vi "Main.vi"(8 "error in":errorcluster, 11 "ArduinoOperator in":refnum<class "ArduinoOperator.lvclass">) -> (0 "error out":errorcluster, 3 "ArduinoOperator out":refnum<class "ArduinoOperator.lvclass">)   [LabVIEW 2018, in "ArduinoOperator.lvclass"]
doc: "The Queued Message Handler of a Worker."
uses:
  ArduinoOperator.lvclass
  Initialization Data.ctl
  <vilib>/addons/_Workers/Library/Classes/Worker/Worker.lvclass
  <vilib>/addons/_Workers/Library/Classes/Message/Message.lvclass
  <vilib>/addons/_Workers/Library/Classes/Message/Enqueue Message to Self v2.vi
  <vilib>/MakerHub/LINX/LMH-LINX.lvlib
  <vilib>/MakerHub/LINX/Public/Utilities/Open Serial.vi
  <vilib>/MakerHub/LINX/Public/Peripherals/Digital/Digital Read 1 Chan.vi
  <vilib>/MakerHub/LINX/Public/Peripherals/Analog/Analog Read 1 Chan.vi
  <vilib>/MakerHub/LINX/Public/Peripherals/Digital/Digital Write 1 Chan.vi
  <vilib>/addons/_Workers/Library/Classes/Message Queue/Message Queue.lvclass
  <vilib>/addons/_Workers/Library/Classes/Message/Priority.ctl
  Timer/Timer.lvclass
  <vilib>/addons/_Workers/Library/Classes/Message/Enqueue Message to Queue.vi
  C:/Program Files (x86)/National Instruments/LabVIEW 2022/vi.lib/addons/_Workers/Library/Classes/Worker/Worker.lvclass
  C:/Program Files (x86)/National Instruments/LabVIEW 2022/vi.lib/addons/_Workers/Library/Classes/Workers Object/Workers Object.lvclass
  <vilib>/addons/_Workers/Library/Classes/Message/Enqueue Message to Self v2 - Silent Mode - Array.vi
panel:
  out "Target":bool
  in  "TimerON":bool
  in  "TimerCount(S)":i32=1
  out "Loop Rate (Hz)":u32
  in  "Close":bool
  in  "Link":bool
  in  "AI Channel":u8
  out "Analog Data":dbl(graph)
  in  "DI Channel":u8=2
  out "DI Value":bool
  in  "DO Value":bool
  in  "DO Channel":u8=3
  in  "Serial Port":refnum<visa-resource-name>
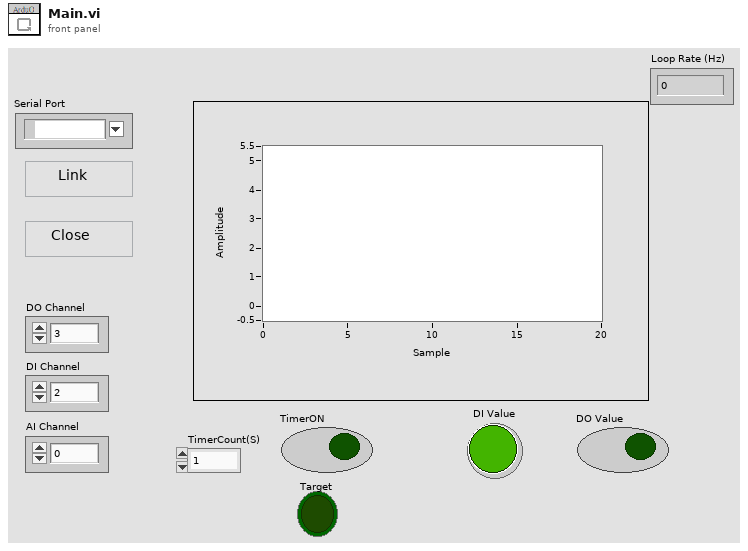
[diagram p1: front panel]
types:
  T1 = typedef "ArduinoOperator.lvclass/Initialization Data.ctl" = cluster{"String":string}
  T2 = typedef "Workers.lvlib/Message.lvclass/Priority.ctl" = enum16{"Low", "Normal", "High"}
  T3 = typedef "Workers.lvlib/Case Label.ctl" = string
  T4 = cluster{"Message Queue out":refnum<class "Message Queue.lvclass">, "Case Label":T3}
  T5 = typedef "LMH-LINX.lvlib/LINX Ref.ctl" = cluster{"IO":T6, "Interface":T7, "LINX Device Config":T8}
  T6 = typedef "LMH-LINX.lvlib/Platform.ctl" = enum16{"Remote", "Local"}
  T7 = typedef "LMH-LINX.lvlib/Interface.ctl" = enum16{"Serial", "TCP"}
  T8 = typedef "LMH-LINX.lvlib/Device.lvlib/LINX Device Config.ctl" = cluster{"Interface":T7, "COM Port":refnum<visa-resource-name>, "TCP Configuration":T9, "Device Family":u8, "Device ID":u8, "Device Name":string, "TCP Ref":refnum<k5>, "Channels":T10}
  T9 = typedef "LMH-LINX.lvlib/Device.lvlib/TCP Config.ctl" = cluster{"IP Address":string, "Port":u16}
  T10 = typedef "LMH-LINX.lvlib/Channels.ctl" = cluster{"DI":u8[], "DO":u8[], "AI":u8[], "AO":u8[], "PWM":u8[], "QE":u8[], "UART":u8[], "I2C 2":u8[], "SPI":u8[], "CAN":u8[], "Servo":u8[], "AI Ref (V)":dbl, "AI Resolution (Bits)":u8, "AO Ref (V)":dbl, "AO Resolution (Bits)":u8}
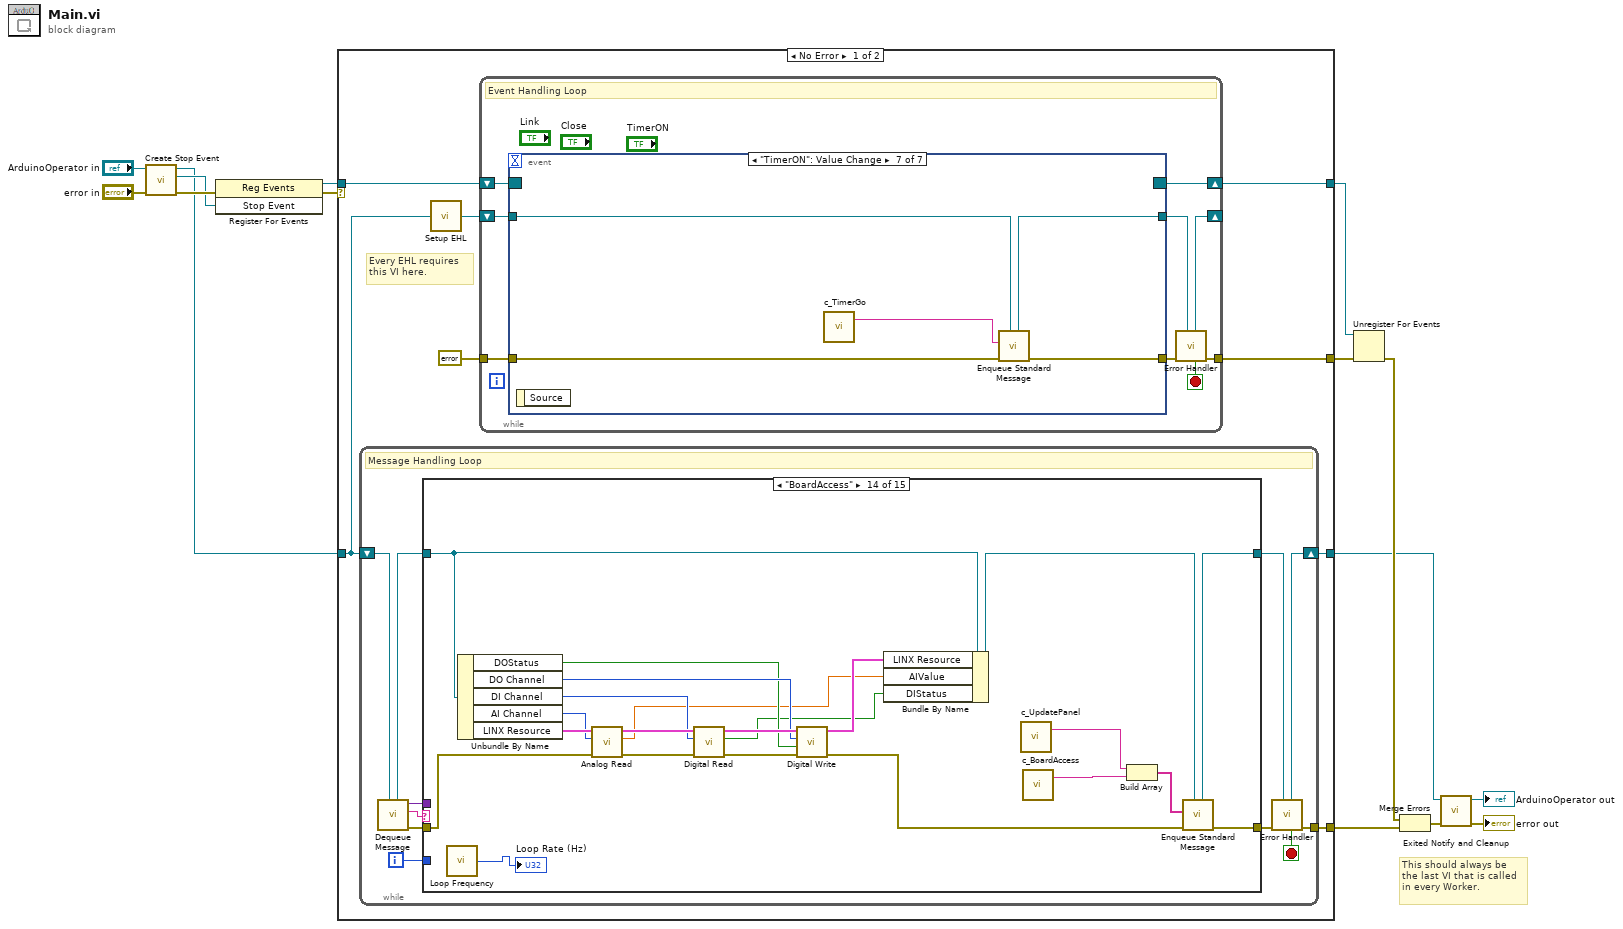
[diagram p0: block diagram]
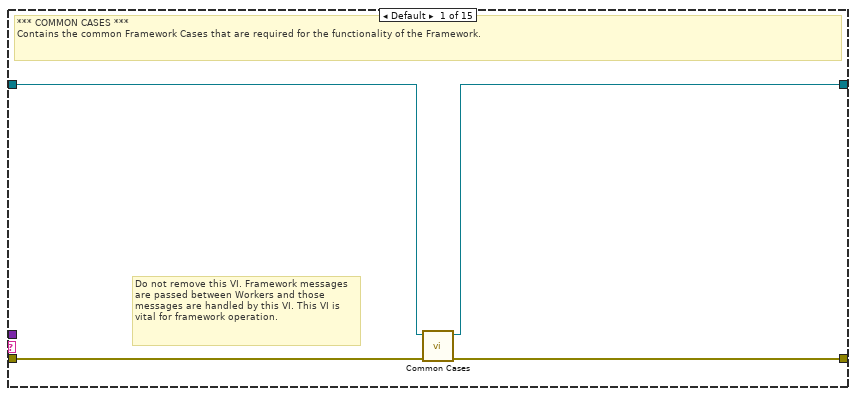
[diagram p2: hidden frame]
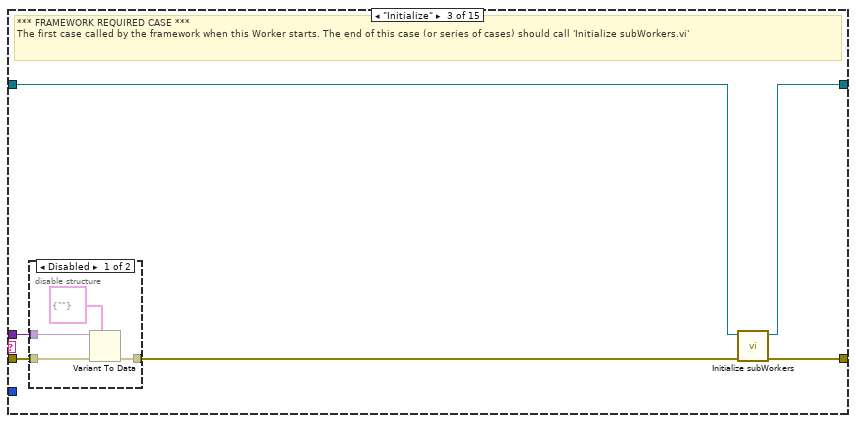
[diagram p4: hidden frame]
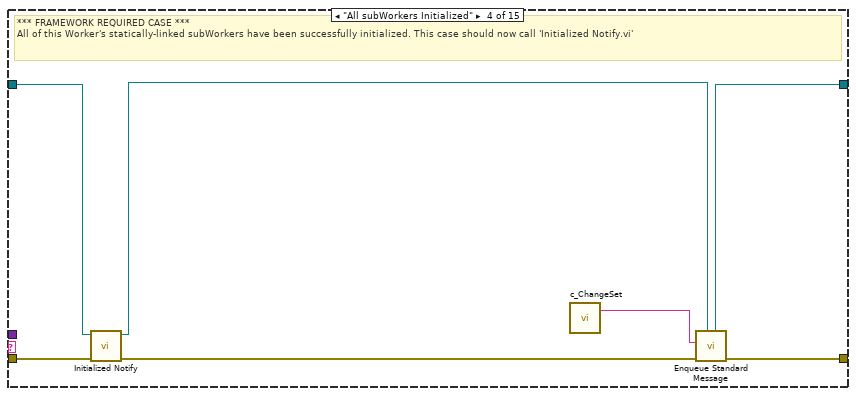
[diagram p6: hidden frame]
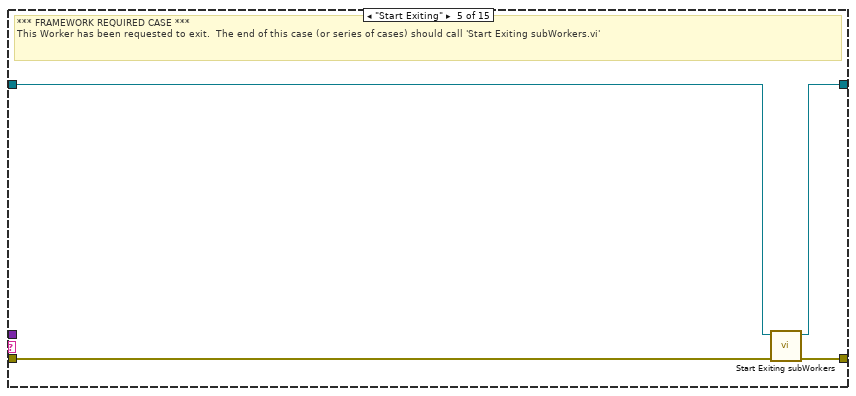
[diagram p7: hidden frame]
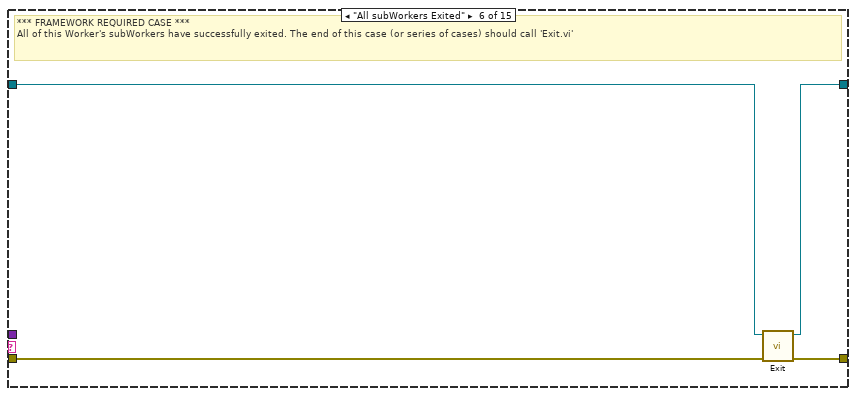
[diagram p8: hidden frame]
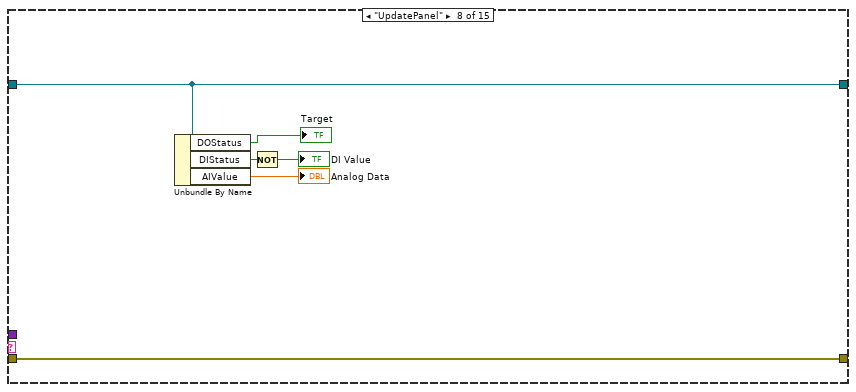
[diagram p10: hidden frame]
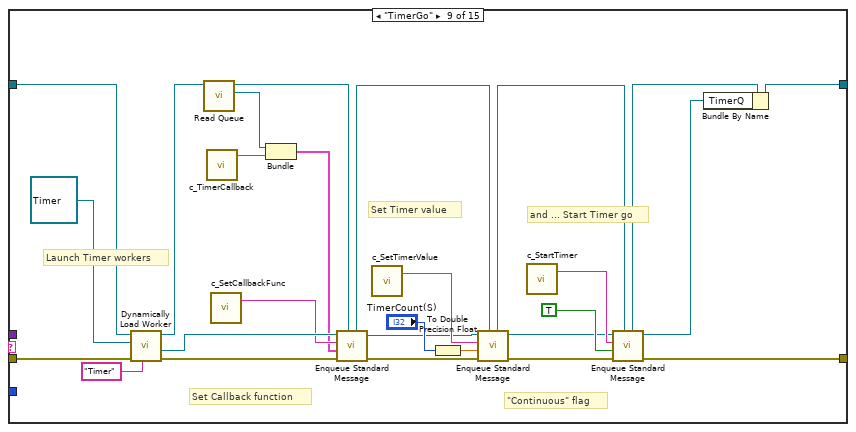
[diagram p11: hidden frame]
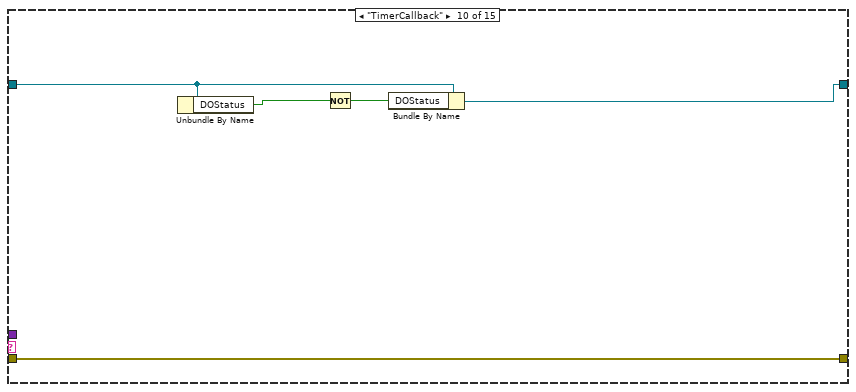
[diagram p12: hidden frame]
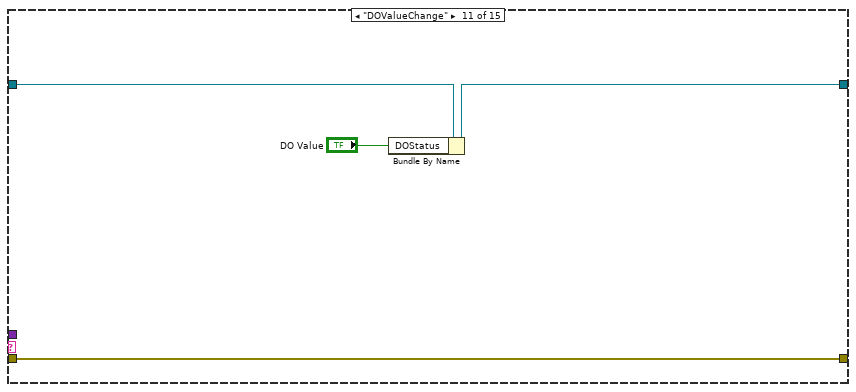
[diagram p13: hidden frame]
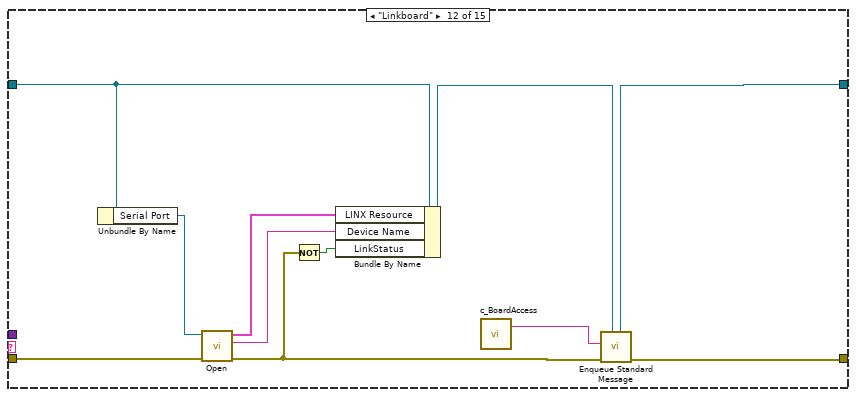
[diagram p14: hidden frame]
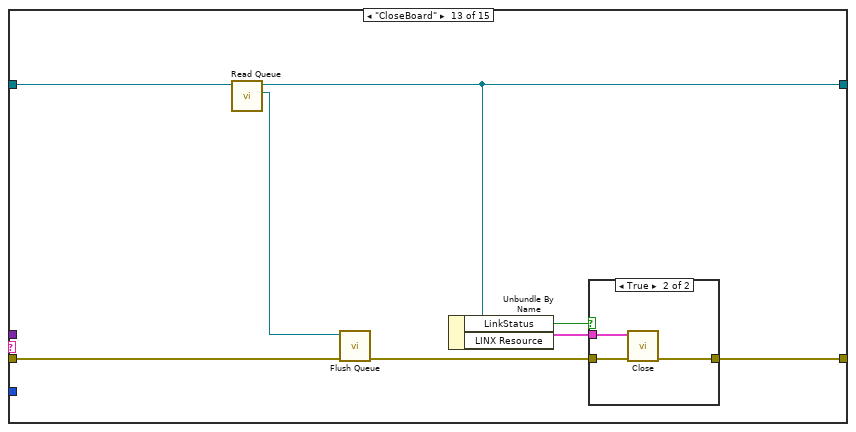
[diagram p15: hidden frame]
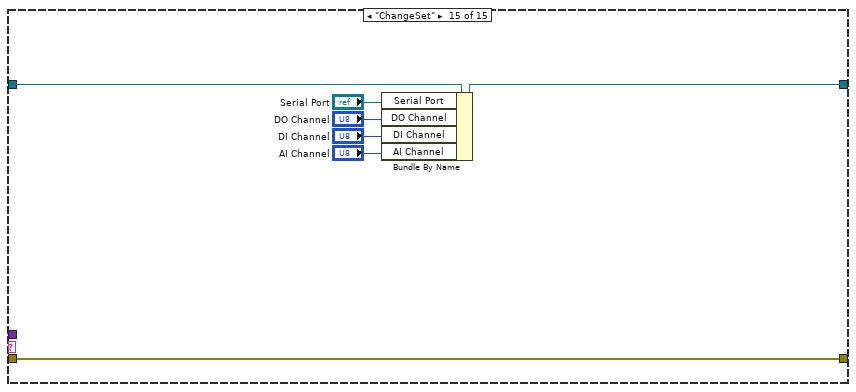
[diagram p17: hidden frame]
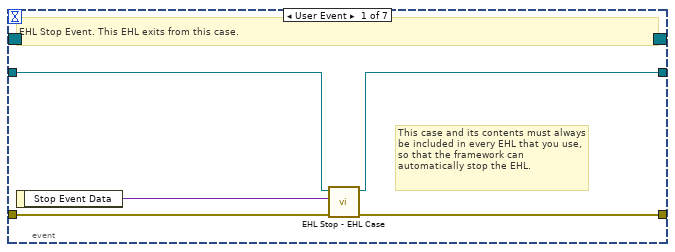
[diagram p18: hidden frame]
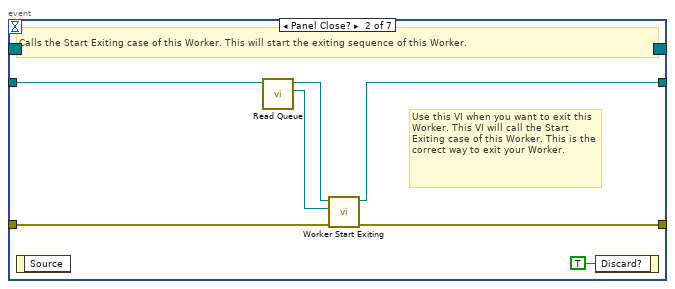
[diagram p19: hidden frame]
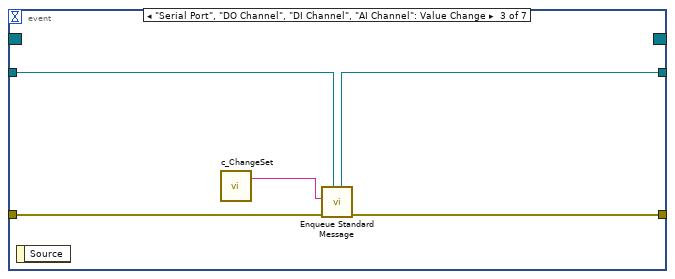
[diagram p20: hidden frame]
diagram:
  # "This should always be the last VI that is called in every Worker."
  n1 = call-dynamic "Create Stop Event.vi"("error in"="error in", "Worker"="ArduinoOperator in") -> ("error out"=w10:errorcluster, "Stop Event"=w7:refnum<user-event>, "Worker out"=w4:refnum<class "ArduinoOperator.lvclass">)  [unwired: 7 in]
  n2 = register-events(error in=w10, w7) -> (reference out=w9:refnum<event-registration>, error out=w1:errorcluster)  [unwired: 1 in]
  n3 = case shown="No Error" w1 {
    tunnel: w4 -> [w18 w211]
    tunnel: [w16 w212] -> w8
    tunnel: w9 -> [w23 w213]
    tunnel: [w20 w214] -> w14
    tunnel: [w22 w213] -> w13
    tunnel: [w17 w210] -> w11
    selector: w1 -> [_ w214]
    frame No Error {
      # "Every EHL requires\nthis VI here."
      n4 = while {
        shift-right: [w32] -> w17
        shift-left: w18 -> [w34]
        tunnel: [w33] -> w16
        i -> [w24]
        stop <- w25 stop-if-true
        # "Message Handling Loop"
        n5 = call-dynamic "Dequeue Message.vi"("Worker"=w34) -> ("error out"=w31:errorcluster, "Case out"=w26:string, "Data out"=w27:variant, "Worker out"=w29:refnum<class "ArduinoOperator.lvclass">)  [unwired: 6 in, 1 out]
        n6 = case "Worker MHL Case Structure (DO NOT CHANGE LABEL NAME)" shown="\"BoardAccess\"" w26 {
          tunnel: w31 -> [w38 w39 w44 w57 w59 w66 w67 w74 w101 w106 w110 w121 w125 w148 w162]
          tunnel: [w37 w39 w46 w55 w62 w65 w67 w74 w93 w106 w110 w113 w126 w138 w162] -> w30
          tunnel: w29 -> [w36 w40 w43 w58 w60 w64 w68 w73 w99 w105 w109 w120 w129 w152 w161]
          tunnel: [w35 w40 w45 w53 w61 w63 w68 w73 w76 w102 w108 w114 w123 w140 w160] -> w28
          tunnel: w27 -> [_ _ w41 _ _ _ _ _ _ _ _ _ _ _ _]
          tunnel: w24 -> [_ _ _ _ _ _ _ _ _ _ _ _ _ _ _]
          frame Default {
            # "Do not remove this VI. Framework messages are passed between Workers and those messages are handled by this VI. This VI is vital for framework operation."
            # "*** COMMON CASES ***\nContains the common Framework Cases that are required for the functionality of the Framework."
            n7 = call-dynamic "Common Cases.vi"("error in"=w38, "Worker in"=w36) -> ("error out"=w37:errorcluster, "Worker out"=w35:refnum<class "ArduinoOperator.lvclass">)  [unwired: 8 in]
          }
          frame "------ FRAMEWORK REQUIRED CASES ------" {
            # "Start of Framework Required Cases"
          }
          frame "Initialize" {
            # "*** FRAMEWORK REQUIRED CASE ***\nThe first case called by the framework when this Worker starts. The end of this case (or series of cases) should call 'Initialize subWorkers.vi'"
            n8 = disable-structure shown="Disabled" {
              disable-tunnel: w44 -> [w50 w51]
              disable-tunnel: [w49 w51] -> w42
              disable-tunnel: w41 -> [w48 _]
              frame Disabled {
                n9 = Variant To Data(error in=w50, type=T1 {"String"=""} ("Initialization Data"), Variant=w48) -> (error out=w49:errorcluster)  [unwired: 1 out]
              }
              frame Enabled {
              }
            }
            n10 = call-dynamic "Initialize subWorkers.vi"("error in"=w42, "Worker"=w43) -> ("error out"=w46:errorcluster, "dup Worker out"=w45:refnum<class "ArduinoOperator.lvclass">)  [unwired: 8 in]
          }
          frame "All subWorkers Initialized" {
            # "*** FRAMEWORK REQUIRED CASE ***\nAll of this Worker's statically-linked subWorkers have been successfully initialized. This case should now call 'Initialized Notify.vi'"
            n11 = call-dynamic "Initialized Notify.vi"("error in"=w57, "Worker"=w58) -> ("error out"=w56:errorcluster, "dup Worker out"=w54:refnum<class "ArduinoOperator.lvclass">)  [unwired: 8 in]
            n12 = call "c_ChangeSet.vi"() -> ("Case Label"=w52:T3)  [unwired: 1 in]
            n13 = call-poly <vilib>:"Enqueue Standard Message.vi"("Worker"=w54, "error in"=w56, "Case Label"=w52) -> ("error out"=w55:errorcluster, "dup Worker out"=w53:refnum<class "ArduinoOperator.lvclass">)  [unwired: 7 in]
          }
          frame "Start Exiting" {
            # "*** FRAMEWORK REQUIRED CASE ***\nThis Worker has been requested to exit.  The end of this case (or series of cases) should call 'Start Exiting subWorkers.vi'"
            n14 = call-dynamic "Start Exiting subWorkers.vi"("error_in"=w59, "Worker"=w60) -> ("error out"=w62:errorcluster, "dup Worker out"=w61:refnum<class "ArduinoOperator.lvclass">)  [unwired: 8 in]
          }
          frame "All subWorkers Exited" {
            # "*** FRAMEWORK REQUIRED CASE ***\nAll of this Worker's subWorkers have successfully exited. The end of this case (or series of cases) should call 'Exit.vi'"
            n15 = call-dynamic "Exit.vi"("error_in"=w66, "Worker"=w64) -> ("error out"=w65:errorcluster, "dup Worker out"=w63:refnum<class "ArduinoOperator.lvclass">)  [unwired: 8 in]
          }
          frame "-----------------------------------------------" {
            # "End of Framework Required Cases"
          }
          frame "UpdatePanel" {
            n16 = Unbundle By Name(w73) -> ("DOStatus"=→"Target":bool, "DIStatus"=w72:bool, "AIValue"=→"Analog Data":dbl)
            n17 = Not(x=w72) -> (.not. x?=→"DI Value":bool)
          }
          frame "TimerGo" {
            # "\"Continuous\" flag"
            # "and ... Start Timer go"
            # "Set Timer value"
            # "Set Callback function"
            # "Launch Timer workers"
            n18 = call <vilib>:"Dynamically Load Worker.vi"("Worker Alias"="Timer", "error in"=w101, "Worker to Dynamically Load"=refnum<class "Timer.lvclass"> refnum ("Timer.lvclass"), "Worker"=w99) -> ("error out"=w100:errorcluster, "Message Queue out"=w84:refnum<class "Message Queue.lvclass">, "dup Worker out"=w86:refnum<class "ArduinoOperator.lvclass">)  [unwired: 4 in, 1 out]
            n19 = call <vilib>:"Read Queue.vi"("Worker"=w86) -> ("Message Queue out"=w79:refnum<class "Message Queue.lvclass">, "dup Worker out"=w81:refnum<class "ArduinoOperator.lvclass">)  [unwired: 9 in]
            n20 = call "c_TimerCallback.vi"() -> ("Case Label"=w80:T3)  [unwired: 1 in]
            n21 = call "c_SetCallbackFunc.vi"() -> ("Case Label"=w82:T3)  [unwired: 1 in]
            n22 = Bundle("Message Queue out"=w79, "Case Label"=w80) -> (w78:T4)  [unwired: 1 in]
            n23 = call-poly <vilib>:"Enqueue Standard Message.vi"("Worker"=w81, "error in"=w100, "Data"=w78, "Case Label"=w82, "Message Queue"=w84) -> ("error out"=w87:errorcluster, "dup Message Queue out"=w83:refnum<class "Message Queue.lvclass">, "dup Worker out"=w85:refnum<class "ArduinoOperator.lvclass">)  [unwired: 4 in]
            n24 = call "c_SetTimerValue.vi"() -> ("Case Label"=w96:T3)  [unwired: 1 in]
            n25 = To Double Precision Float(number="TimerCount(S)") -> (double precision float=w94:dbl)
            n26 = call-poly <vilib>:"Enqueue Standard Message.vi"("Worker"=w85, "error in"=w87, "Data"=w94, "Case Label"=w96, "Message Queue"=w83) -> ("error out"=w97:errorcluster, "dup Message Queue out"=w77:refnum<class "Message Queue.lvclass">, "dup Worker out"=w92:refnum<class "ArduinoOperator.lvclass">)  [unwired: 4 in]
            n27 = call "c_StartTimer.vi"() -> ("Case Label"=w90:T3)  [unwired: 1 in]
            n28 = call-poly <vilib>:"Enqueue Standard Message.vi"("Worker"=w92, "error in"=w97, "Data"=TRUE, "Case Label"=w90, "Message Queue"=w77) -> ("error out"=w93:errorcluster, "dup Message Queue out"=w75:refnum<class "Message Queue.lvclass">, "dup Worker out"=w91:refnum<class "ArduinoOperator.lvclass">)  [unwired: 4 in]
            n29 = Bundle By Name(cluster=w91, "TimerQ"=w75) -> (w76:refnum<class "ArduinoOperator.lvclass">)
          }
          frame "TimerCallback" {
            n30 = Unbundle By Name(w105) -> ("DOStatus"=w104:bool)
            n31 = Not(x=w104) -> (.not. x?=w103:bool)
            n32 = Bundle By Name(cluster=w105, "DOStatus"=w103) -> (w102:refnum<class "ArduinoOperator.lvclass">)
          }
          frame "DOValueChange" {
            n33 = Bundle By Name(cluster=w109, "DOStatus"="DO Value") -> (w108:refnum<class "ArduinoOperator.lvclass">)
          }
          frame "Linkboard" {
            n34 = Unbundle By Name(w120) -> ("Serial Port"=w119:refnum<visa-resource-name>)
            n35 = call-poly <vilib>:"Open.vi"("Error In"=w121, "Serial Port"=w119) -> ("Error Out"=w112:errorcluster, "Device Name"=w116:string, "LINX Resource"=w117:T5)  [unwired: 7 in]
            n36 = Not(x=w112) -> (.not. x?=w115:bool)
            n37 = Bundle By Name(cluster=w120, "LINX Resource"=w117, "Device Name"=w116, "LinkStatus"=w115) -> (w118:refnum<class "ArduinoOperator.lvclass">)
            n38 = call "c_BoardAccess.vi"() -> ("Case Label"=w111:T3)  [unwired: 1 in]
            n39 = call-poly <vilib>:"Enqueue Standard Message.vi"("Worker"=w118, "error in"=w112, "Case Label"=w111) -> ("error out"=w113:errorcluster, "dup Worker out"=w114:refnum<class "ArduinoOperator.lvclass">)  [unwired: 7 in]
          }
          frame "CloseBoard" {
            n40 = call <vilib>:"Read Queue.vi"("Worker"=w129) -> ("Message Queue out"=w122:refnum<class "Message Queue.lvclass">, "dup Worker out"=w123:refnum<class "ArduinoOperator.lvclass">)  [unwired: 9 in]
            n41 = call <vilib>:"Flush Queue.vi"("error in (no error)"=w125, "Message Queue"=w122) -> ("error out"=w124:errorcluster)  [unwired: 7 in, 2 out]
            n42 = Unbundle By Name(w123) -> ("LinkStatus"=w127:bool, "LINX Resource"=w128:T5)
            n43 = case shown="True" w127 {
              tunnel: w128 -> [_ w133]
              tunnel: w124 -> [w130 w132]
              tunnel: [w130 w131] -> w126
              frame False {
              }
              frame True {
                n44 = call <vilib>:"Close.vi"("Error In"=w132, "LINX Resource"=w133) -> ("Error Out"=w131:errorcluster)  [unwired: 9 in]
              }
            }
          }
          frame "BoardAccess" {
            n45 = call <vilib>:"Loop Frequency.vi"() -> ("Loop Rate (Hz)"=→"Loop Rate (Hz)":u32)
            n46 = Unbundle By Name(w152) -> ("DOStatus"=w145:bool, "DO Channel"=w146:u8, "DI Channel"=w147:u8, "AI Channel"=w151:u8, "LINX Resource"=w153:T5)
            n47 = call-poly <vilib>:"Analog Read.vi"("Error In"=w148, "Analog Channel"=w151, "LINX Resource"=w153) -> ("Error Out"=w155:errorcluster, "Voltage"=w142:dbl, "LINX Resource"=w150:T5)  [unwired: 5 in, 1 out]
            n48 = call-poly <vilib>:"Digital Read.vi"("Error In"=w155, "DI Channel"=w147, "LINX Resource"=w150) -> ("Error Out"=w154:errorcluster, "DI Value"=w141:bool, "LINX Resource"=w149:T5)  [unwired: 6 in]
            n49 = call-poly <vilib>:"Digital Write.vi"("Error In"=w154, "Output Value"=w145, "DO Channel"=w146, "LINX Resource"=w149) -> ("Error Out"=w139:errorcluster, "LINX Resource"=w143:T5)  [unwired: 6 in]
            n50 = Bundle By Name(cluster=w152, "LINX Resource"=w143, "AIValue"=w142, "DIStatus"=w141) -> (w144:refnum<class "ArduinoOperator.lvclass">)
            n51 = call "c_UpdatePanel.vi"() -> ("Case Label"=w136:T3)  [unwired: 1 in]
            n52 = call "c_BoardAccess.vi"() -> ("Case Label"=w135:T3)  [unwired: 1 in]
            n53 = Build Array(w136, w135) -> (w134:T3[])
            n54 = call-poly <vilib>:"Enqueue Standard Message.vi"("Worker"=w144, "error in"=w139, "Case Label []"=w134) -> ("error out"=w138:errorcluster, "dup Worker out"=w140:refnum<class "ArduinoOperator.lvclass">)  [unwired: 7 in]
          }
          frame "ChangeSet" {
            n55 = Bundle By Name(cluster=w161, "Serial Port"="Serial Port", "DO Channel"="DO Channel", "DI Channel"="DI Channel", "AI Channel"="AI Channel") -> (w160:refnum<class "ArduinoOperator.lvclass">)
          }
        }
        n56 = call-dynamic "Error Handler.vi"("Worker"=w28, "error_in"=w30) -> ("error out"=w33:errorcluster, "Stop Loop"=w25:bool, "Worker out"=w32:refnum<class "ArduinoOperator.lvclass">)  [unwired: 7 in]
      }
      n57 = call-dynamic "Setup EHL.vi"("Worker"=w18) -> ("Worker out"=w19:refnum<class "ArduinoOperator.lvclass">)  [unwired: 14 in]
      n58 = while "Event Handling Loop" {
        shift-right: [w171] -> w22
        shift-left: w23 -> [w170]
        tunnel: [w166] -> w20
        tunnel: errorcluster {"status"=FALSE, "code"=0, "source"=""} ("error constant") -> [w168]
        shift-right: [w164] -> _
        shift-left: w19 -> [w169]
        stop <- w163 stop-if-true
        # "Event Handling Loop"
        n59 = event shown="[6] \"TimerON\": Value Change" {
          selector: w170 -> [_ _ _ _ _ _ _]
          dyn-events: [_ _ _ _ _ _ _] -> w171
          timeout: _ -> [_ _ _ _ _ _ _]
          tunnel: [w175 w182 w187 w193 w198 w203 w208] -> w167
          tunnel: w168 -> [w176 w181 w188 w194 w199 w204 w209]
          tunnel: w169 -> [w174 w180 w186 w192 w197 w202 w207]
          tunnel: [w173 w179 w185 w191 w196 w201 w206] -> w165
          event User Event {
            # "This case and its contents must always be included in every EHL that you use, so that the framework can automatically stop the EHL."
            # "EHL Stop Event. This EHL exits from this case."
            n60 = event-data() -> ("Stop Event Data"=w172:variant)  [unwired: 1 in]
            n61 = call <vilib>:"EHL Stop - EHL Case.vi"("error in"=w176, "Stop Event Data"=w172, "Worker"=w174) -> ("error out"=w175:errorcluster, "Worker out"=w173:refnum<class "ArduinoOperator.lvclass">)  [unwired: 7 in]
          }
          event Panel Close? {
            # "Use this VI when you want to exit this Worker. This VI will call the Start Exiting case of this Worker. This is the correct way to exit your Worker."
            # "Calls the Start Exiting case of this Worker. This will start the exiting sequence of this Worker."
            n62 = event-data() -> ()  [unwired: 1 in, 1 out]
            n63 = call <vilib>:"Read Queue.vi"("Worker"=w180) -> ("Message Queue out"=w177:refnum<class "Message Queue.lvclass">, "dup Worker out"=w178:refnum<class "ArduinoOperator.lvclass">)  [unwired: 9 in]
            n64 = call-dynamic "Worker Start Exiting.vi"("error_in"=w181, "Message Queue"=w177, "Worker"=w178) -> ("error out"=w182:errorcluster, "dup Worker out"=w179:refnum<class "ArduinoOperator.lvclass">)  [unwired: 7 in]
            n65 = event-data("Discard?"=TRUE) -> ()  [unwired: 1 in, 1 out]
          }
          event "Serial Port", "DO Channel", "DI Channel", "AI Channel": Value Change {
            n66 = event-data() -> ()  [unwired: 1 in, 1 out]
            n67 = call "c_ChangeSet.vi"() -> ("Case Label"=w184:T3)  [unwired: 1 in]
            n68 = call-poly <vilib>:"Enqueue Standard Message.vi"("Worker"=w186, "error in"=w188, "Case Label"=w184) -> ("error out"=w187:errorcluster, "dup Worker out"=w185:refnum<class "ArduinoOperator.lvclass">)  [unwired: 7 in]
          }
          event "DO Value": Value Change {
            n69 = event-data() -> ()  [unwired: 1 in, 1 out]
            n70 = call "c_DOValueChange.vi"() -> ("Case Label"=w190:T3)  [unwired: 1 in]
            n71 = call-poly <vilib>:"Enqueue Standard Message.vi"("Priority (Normal)"=Priority."High", "Worker"=w192, "error in"=w194, "Case Label"=w190) -> ("error out"=w193:errorcluster, "dup Worker out"=w191:refnum<class "ArduinoOperator.lvclass">)  [unwired: 6 in]
          }
          event "Link": Value Change {
            n72 = event-data() -> ()  [unwired: 1 in, 1 out]
            n73 = call "c_Linkboard.vi"() -> ("Case Label"=w195:T3)  [unwired: 1 in]
            n74 = call-poly <vilib>:"Enqueue Standard Message.vi"("Worker"=w197, "error in"=w199, "Case Label"=w195) -> ("error out"=w198:errorcluster, "dup Worker out"=w196:refnum<class "ArduinoOperator.lvclass">)  [unwired: 7 in]
          }
          event "Close": Value Change {
            n75 = event-data() -> ()  [unwired: 1 in, 1 out]
            n76 = call "c_CloseBoard.vi"() -> ("Case Label"=w200:T3)  [unwired: 1 in]
            n77 = call-poly <vilib>:"Enqueue Standard Message.vi"("Worker"=w202, "error in"=w204, "Case Label"=w200) -> ("error out"=w203:errorcluster, "dup Worker out"=w201:refnum<class "ArduinoOperator.lvclass">)  [unwired: 7 in]
          }
          event "TimerON": Value Change {
            n78 = event-data() -> ()  [unwired: 1 in, 1 out]
            n79 = call "c_TimerGo.vi"() -> ("Case Label"=w205:T3)  [unwired: 1 in]
            n80 = call-poly <vilib>:"Enqueue Standard Message.vi"("Worker"=w207, "error in"=w209, "Case Label"=w205) -> ("error out"=w208:errorcluster, "dup Worker out"=w206:refnum<class "ArduinoOperator.lvclass">)  [unwired: 7 in]
          }
        }
        n81 = call-dynamic "Error Handler.vi"("Worker"=w165, "error_in"=w167) -> ("error out"=w166:errorcluster, "Stop Loop"=w163:bool, "Worker out"=w164:refnum<class "ArduinoOperator.lvclass">)  [unwired: 7 in]
      }
    }
    frame Error {
      n82 = call-dynamic "Error Handler.vi"("Worker"=w211, "error_in"=w214) -> ("error out"=w212:errorcluster, "Worker out"=w210:refnum<class "ArduinoOperator.lvclass">)  [unwired: 7 in, 1 out]
    }
  }
  n83 = Unregister For Events(event registration refnum=w13, error in=w14) -> (error out=w15:errorcluster)
  n84 = Merge Errors(w15, w8) -> (w12:errorcluster)
  n85 = call-dynamic "Exited Notify and Cleanup.vi"("error_in"=w12, "Worker"=w11) -> ("error out"=→"error out":errorcluster, "dup Worker out"=→"ArduinoOperator out":refnum<class "ArduinoOperator.lvclass">)  [unwired: 8 in]
